vi "getData.vi"(11 "Local Debug":bool) -> ()   [LabVIEW 2017]
uses:
  <vilib>/httpClient/ClientHandle.ctl
  msg7171_linux.llb/send single message.vi
  msg7171_linux.llb/send multiple messages.vi
  <vilib>/httpClient/LabVIEWHTTPClient.lvlib
panel:
  in  "exit":bool
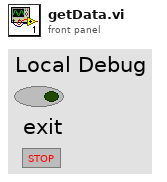
[diagram p1: front panel]
types:
  T1 = typedef "LabVIEWHTTPClient.lvlib/ClientHandle.ctl" = refnum<k1>
  T2 = cluster{"go":bool, "Http session":T1, "URL prefex":string}
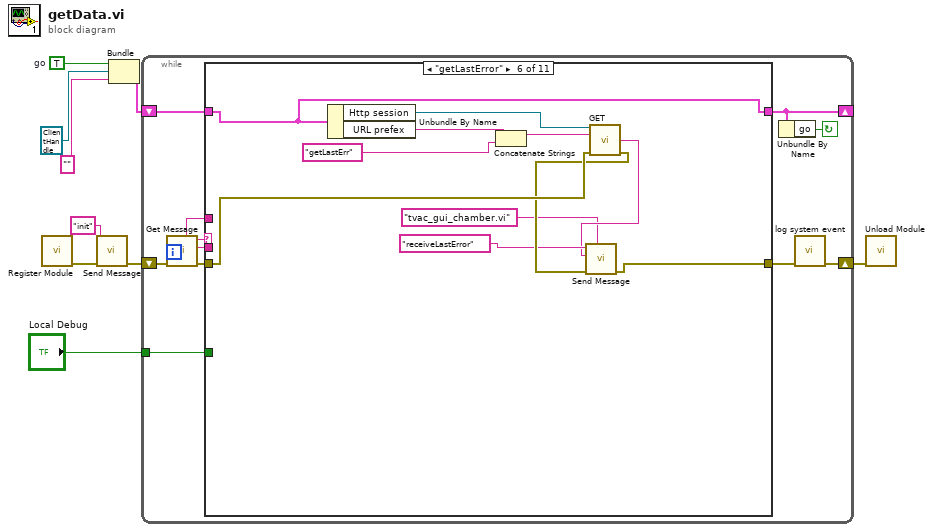
[diagram p0: block diagram]
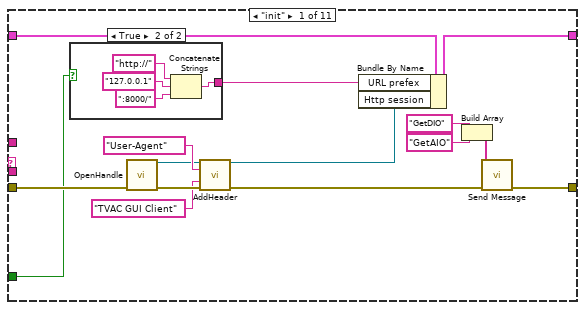
[diagram p2: hidden frame]
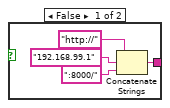
[diagram p3: hidden frame]
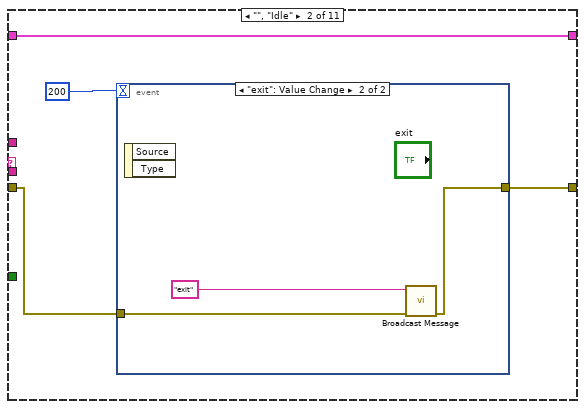
[diagram p4: hidden frame]
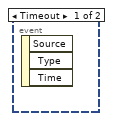
[diagram p5: hidden frame]
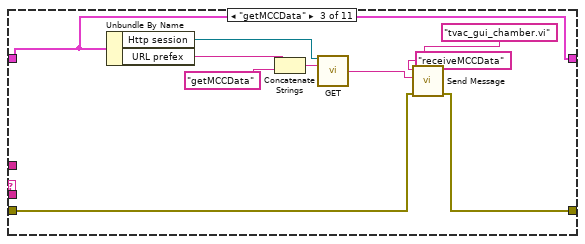
[diagram p6: hidden frame]
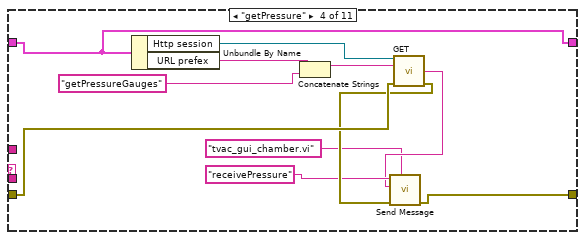
[diagram p7: hidden frame]
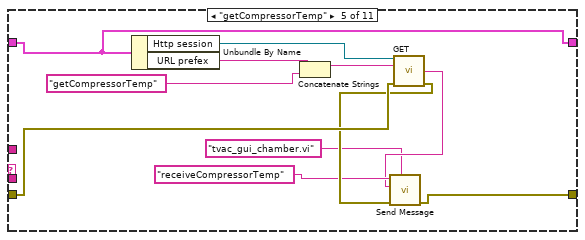
[diagram p8: hidden frame]
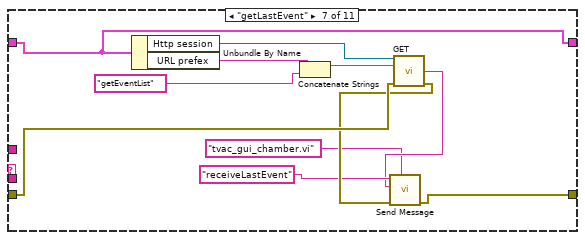
[diagram p9: hidden frame]
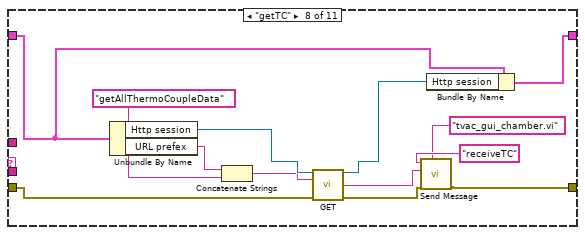
[diagram p10: hidden frame]
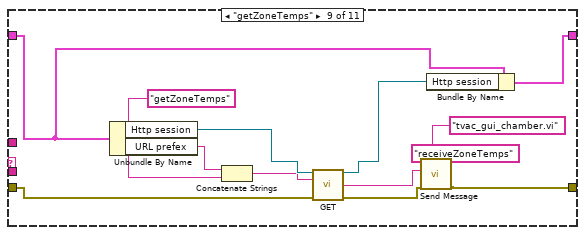
[diagram p11: hidden frame]
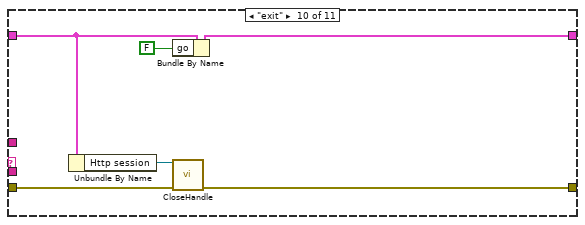
[diagram p12: hidden frame]
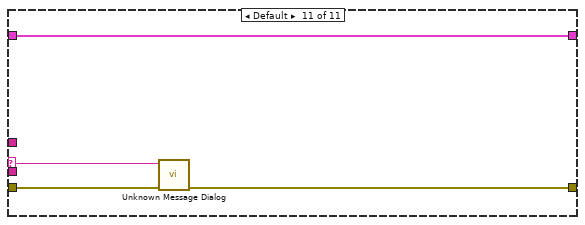
[diagram p13: hidden frame]
diagram:
  w7 = TRUE  # go
  n1 = call "Register Module.vi"() -> ("error out"=w3:errorcluster)  [unwired: 10 in, 1 out]
  n2 = call-poly "Send Message.vi"("error in (no error)"=w3, "event"="init") -> ("error out"=w2:errorcluster)  [unwired: 9 in]
  n3 = Bundle("go"=w7, "Http session"=T1 refnum, "URL prefex"="") -> (w9:T2)  [unwired: 1 in]
  n4 = while {
    shift-left: w9 -> [w17]
    shift-right: [w15] -> _
    shift-right: [w13] -> w8
    shift-left: w2 -> [w20]
    tunnel: "Local Debug" -> [w10]
    stop <- w14 continue-if-true
    n5 = call "Get Message.vi"("error in (no error)"=w20) -> ("error out"=w18:errorcluster, "event buffer"=w19:string, "event"=w16:string, "source"=w11:string)  [unwired: 7 in]
    n6 = case shown="\"getLastError\"" w16 {
      selector: w16 -> [_ _ _ _ _ _ _ _ _ _ w138]
      tunnel: [w29 w45 w55 w61 w72 w83 w94 w111 w124 w136 w140] -> w15
      tunnel: w17 -> [w35 w45 w55 w61 w72 w83 w94 w113 w126 w131 w140]
      tunnel: w19 -> [_ _ _ _ _ _ _ _ _ _ _]
      tunnel: w18 -> [w30 w47 w57 w67 w78 w89 w100 w114 w127 w134 w139]
      tunnel: [w25 w46 w56 w65 w76 w87 w98 w109 w122 w133 w137] -> w12
      tunnel: w11 -> [_ _ _ _ _ _ _ _ _ _ _]
      tunnel: w10 -> [w21 _ _ _ _ _ _ _ _ _ _]
      frame "init" {
        n7 = case shown="True" w21 {
          tunnel: [w36 w41] -> w28
          frame False {
            n8 = Concatenate Strings("http://" ("url"), "192.168.99.1" ("Address"), ":8000/" ("url")) -> (w36:string)
          }
          frame True {
            n9 = Concatenate Strings("http://" ("url"), "127.0.0.1" ("Address"), ":8000/" ("url")) -> (w41:string)
          }
        }
        n10 = call <vilib>:"OpenHandle.vi"("error in (no error)"=w30) -> ("client handle out"=w31:T1, "error out"=w34:errorcluster)  [unwired: 13 in]
        n11 = call <vilib>:"AddHeader.vi"("client handle"=w31, "header"="User-Agent", "value"="TVAC GUI Client", "error in (no error)"=w34) -> ("client handle out"=w27:T1, "error out"=w26:errorcluster)  [unwired: 10 in]
        n12 = Bundle By Name(cluster=w35, "URL prefex"=w28, "Http session"=w27) -> (w29:T2)
        n13 = Build Array("GetDIO" ("event"), "GetAIO" ("event")) -> (w23:string[])
        n14 = call-poly "Send Message.vi"("error in (no error)"=w26, "event"=w23) -> ("error out"=w25:errorcluster)  [unwired: 9 in]
      }
      frame "", "Idle" {
        n15 = event shown="[1] \"exit\": Value Change" {
          selector: _ -> [_ _]
          dyn-events: _ -> [_ _]
          timeout: 200 ("Numeric") -> [_ _]
          tunnel: w47 -> [_ w49]
          tunnel: [_ w48] -> w46
          event Timeout {
            n16 = event-data() -> ()  [unwired: 1 in, 3 out]
          }
          event "exit": Value Change {
            n17 = event-data() -> ()  [unwired: 1 in, 2 out]
            n18 = call "Broadcast Message.vi"("error in (no error)"=w49, "event"="exit") -> ("error out"=w48:errorcluster)  [unwired: 9 in]
          }
        }
      }
      frame "getMCCData" {
        n19 = Unbundle By Name(w55) -> ("Http session"=w51:T1, "URL prefex"=w53:string)
        n20 = Concatenate Strings(w53, "getMCCData" ("url")) -> (w54:string)
        n21 = call <vilib>:"GET.vi"("client handle"=w51, "url"=w54) -> ("body"=w59:string)  [unwired: 10 in, 3 out]
        n22 = call-poly "Send Message.vi"("Destination Module"="tvac_gui_chamber.vi", "error in (no error)"=w57, "event buffer"=w59, "event"="receiveMCCData" ("url")) -> ("error out"=w56:errorcluster)  [unwired: 7 in]
      }
      frame "getPressure" {
        n23 = Unbundle By Name(w61) -> ("Http session"=w68:T1, "URL prefex"=w70:string)
        n24 = Concatenate Strings(w70, "getPressureGauges" ("url")) -> (w71:string)
        n25 = call <vilib>:"GET.vi"("client handle"=w68, "url"=w71, "error in (no error)"=w67) -> ("body"=w63:string, "error out"=w66:errorcluster)  [unwired: 9 in, 2 out]
        n26 = call-poly "Send Message.vi"("Destination Module"="tvac_gui_chamber.vi", "error in (no error)"=w66, "event buffer"=w63, "event"="receivePressure" ("url")) -> ("error out"=w65:errorcluster)  [unwired: 7 in]
      }
      frame "getCompressorTemp" {
        n27 = Unbundle By Name(w72) -> ("Http session"=w79:T1, "URL prefex"=w81:string)
        n28 = Concatenate Strings(w81, "getCompressorTemp" ("url")) -> (w82:string)
        n29 = call <vilib>:"GET.vi"("client handle"=w79, "url"=w82, "error in (no error)"=w78) -> ("body"=w74:string, "error out"=w77:errorcluster)  [unwired: 9 in, 2 out]
        n30 = call-poly "Send Message.vi"("Destination Module"="tvac_gui_chamber.vi", "error in (no error)"=w77, "event buffer"=w74, "event"="receiveCompressorTemp" ("url")) -> ("error out"=w76:errorcluster)  [unwired: 7 in]
      }
      frame "getLastError" {
        n31 = Unbundle By Name(w83) -> ("Http session"=w90:T1, "URL prefex"=w92:string)
        n32 = Concatenate Strings(w92, "getLastErr" ("url")) -> (w93:string)
        n33 = call <vilib>:"GET.vi"("client handle"=w90, "url"=w93, "error in (no error)"=w89) -> ("body"=w85:string, "error out"=w88:errorcluster)  [unwired: 9 in, 2 out]
        n34 = call-poly "Send Message.vi"("Destination Module"="tvac_gui_chamber.vi", "error in (no error)"=w88, "event buffer"=w85, "event"="receiveLastError" ("url")) -> ("error out"=w87:errorcluster)  [unwired: 7 in]
      }
      frame "getLastEvent" {
        n35 = Unbundle By Name(w94) -> ("Http session"=w101:T1, "URL prefex"=w103:string)
        n36 = Concatenate Strings(w103, "getEventList" ("url")) -> (w104:string)
        n37 = call <vilib>:"GET.vi"("client handle"=w101, "url"=w104, "error in (no error)"=w100) -> ("body"=w96:string, "error out"=w99:errorcluster)  [unwired: 9 in, 2 out]
        n38 = call-poly "Send Message.vi"("Destination Module"="tvac_gui_chamber.vi", "error in (no error)"=w99, "event buffer"=w96, "event"="receiveLastEvent" ("url")) -> ("error out"=w98:errorcluster)  [unwired: 7 in]
      }
      frame "getTC" {
        n39 = Unbundle By Name(w113) -> ("Http session"=w117:T1, "URL prefex"=w105:string)
        n40 = Concatenate Strings(w105, "getAllThermoCoupleData" ("url")) -> (w116:string)
        n41 = call <vilib>:"GET.vi"("client handle"=w117, "url"=w116, "error in (no error)"=w114) -> ("client handle out"=w112:T1, "body"=w107:string, "error out"=w110:errorcluster)  [unwired: 9 in, 1 out]
        n42 = call-poly "Send Message.vi"("Destination Module"="tvac_gui_chamber.vi", "error in (no error)"=w110, "event buffer"=w107, "event"="receiveTC" ("url")) -> ("error out"=w109:errorcluster)  [unwired: 7 in]
        n43 = Bundle By Name(cluster=w113, "Http session"=w112) -> (w111:T2)
      }
      frame "getZoneTemps" {
        n44 = Unbundle By Name(w126) -> ("Http session"=w130:T1, "URL prefex"=w118:string)
        n45 = Concatenate Strings(w118, "getZoneTemps" ("url")) -> (w129:string)
        n46 = call <vilib>:"GET.vi"("client handle"=w130, "url"=w129, "error in (no error)"=w127) -> ("client handle out"=w125:T1, "body"=w120:string, "error out"=w123:errorcluster)  [unwired: 9 in, 1 out]
        n47 = call-poly "Send Message.vi"("Destination Module"="tvac_gui_chamber.vi", "error in (no error)"=w123, "event buffer"=w120, "event"="receiveZoneTemps" ("url")) -> ("error out"=w122:errorcluster)  [unwired: 7 in]
        n48 = Bundle By Name(cluster=w126, "Http session"=w125) -> (w124:T2)
      }
      frame "exit" {
        n49 = Unbundle By Name(w131) -> ("Http session"=w132:T1)
        n50 = Bundle By Name(cluster=w131, "go"=FALSE ("Bundle Element")) -> (w136:T2)
        n51 = call <vilib>:"CloseHandle.vi"("client handle"=w132, "error in (no error)"=w134) -> ("error out"=w133:errorcluster)  [unwired: 13 in]
      }
      frame Default {
        n52 = call "Unknown Message Dialog.vi"("error in (no error)"=w139, "event name"=w138) -> ("error out"=w137:errorcluster)  [unwired: 9 in]
      }
    }
    n53 = Unbundle By Name(w15) -> ("go"=w14:bool)
    n54 = call "log system event.vi"("error in (no error)"=w12) -> ("error out"=w13:errorcluster)  [unwired: 9 in, 1 out]
  }
  n55 = call "Unload Module.vi"("error in (no error)"=w8) -> ()  [unwired: 10 in, 1 out]
